vi "Multi-Record Stream Control.vi"(0 "actual state from slave":T1, 1 "ready to restart":bool, 2 "request state":T1, 3 "samples transferred":u64, 4 "num records":u64, 8 "reset":bool) -> (14 "request state to slave":T1, 15 "request to restart":bool, 16 "actual state":T1, 17 "total samples transferred":u64)   [LabVIEW 2018, in "Streaming FPGA.lvlib"]
doc: "Extends the <B>Acquisition Stream Control.vi</B> and the <B>Generation Stream Control.vi</B> with multi-record functionality.\n\nA finite transfer can be started by commanding the stream control VI from the \"Idle\" state to the \"Finite Transfer\" state. After the specified number of samples are transferred, the stream control VI enters the \"Done\" state. This multi-record stream control VI controls and monitors the state of a stream control VI to repeat the finite transfer <B>num records</B> times.\n\nThe <B>request state</B> input of this VI should receive the desired state of the multi-record stream control and the <B>request state to slave</B> output of this VI should drive the <B>request state</B> input of the stream control (<B>Acquisition Stream Control.vi</B> or <B>Generation Stream Control.vi</B>). Connect the <B>actual state</B> and <B>samples transferred</B> outputs of the stream control to the <B>actual state from slave</B> and <B>samples transferred</B> inputs of this VI through a Feedback Node. The <B>actual state</B> output of this VI returns the state of the multi-record stream control while the <B>total samples transferred</B> returns the total number of samples transferred since the multi-record transfer was started.\n\nCommanding the multi-record stream control from the \"Idle\" to the \"Finite Transfer\" state starts the multi-record transfer of <B>num records</B> records. For each record, the stream control is commanded from the \"Idle\" to the \"Finite Transfer\" state. When the stream control enters the \"Done\" state (signaling that the finite transfer is complete) and there are more records, the <B>request to restart</B> output is set to true for one cycle and the stream control is commanded into the \"Idle\" state, and a wait of 4 clock cycles starts. Once the wait is complete and the stream control enters the \"Idle\" state and a true is detected on the <B>ready to restart</B> input, the transfer of the next record starts by commanding the stream control from the \"Idle\" to the \"Finite Transfer\" state. During the multi-record transfer the <B>actual state</B> output returns \"Finite Transfer\" if the stream control indicates normal operation. If the stream control indicates an error or if a different state is requested on the <B>request state</B> input, then the multi-record transfer stops. When the stream control enters the \"Done\" state (signaling that the finite transfer is complete) and there are no more records, this VI also enters the \"Done\" state.\n\nWhen no multi-record transfer is in progress, the <B>request state to slave</B> output returns the <B>request state</B> input while the <B>actual state</B> and <B>total samples transferred</B> outputs return the <B>actual state from slave</B> and <B>samples transferred</B> inputs."
uses:
  Streaming FPGA.lvlib
  <instrlib>/_niInstr/Streaming/v1/Common/Stream State.ctl
  <instrlib>/_niInstr/Streaming/v1/Common/niInstr Streaming v1 Common.lvlib
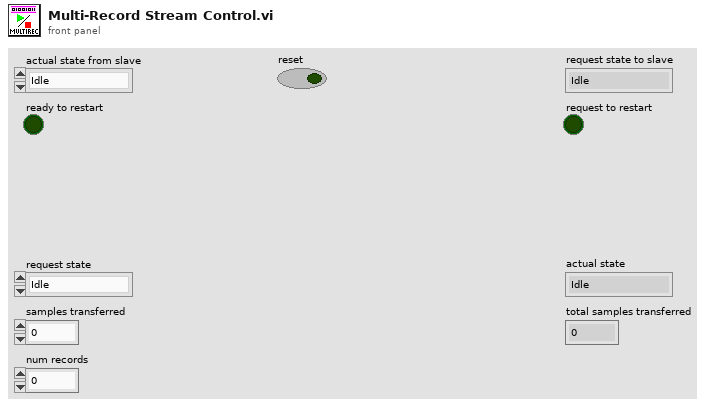
[diagram p1: front panel]
types:
  T1 = typedef "niInstr Streaming v1 Common.lvlib/Stream State.ctl" = enum8{"Idle", "Finite Transfer", "Continuous", "Done", "Error", "Not Ready", "Cancel"}
  T2 = enum16{"Idle", "Start Record", "Wait For Done", "Wait For Idle"}
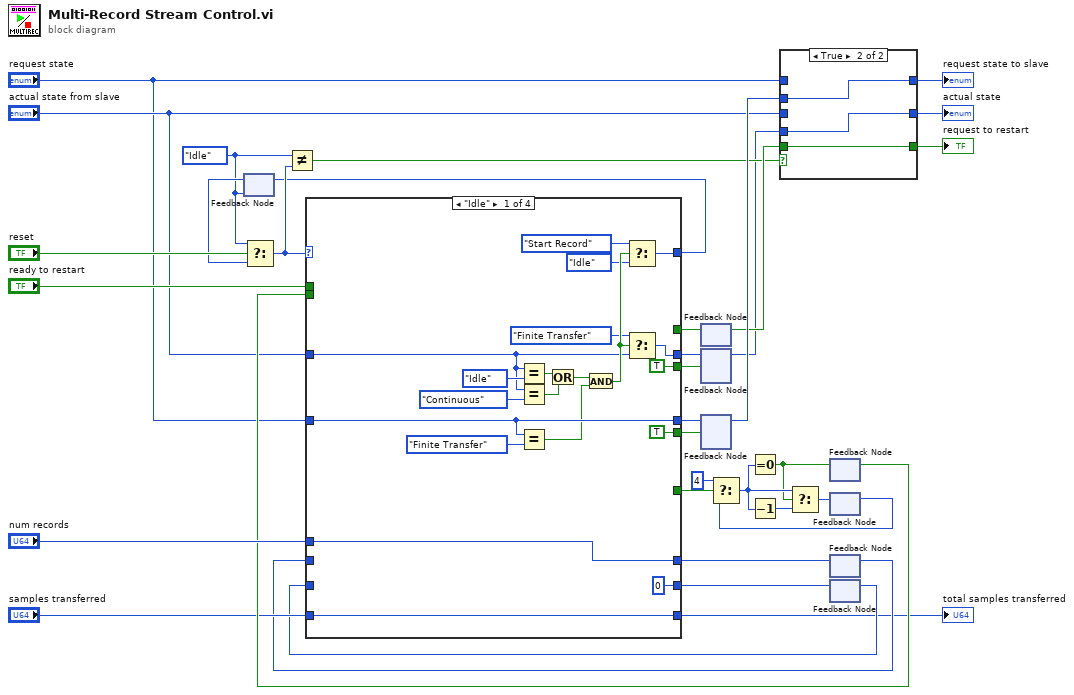
[diagram p0: block diagram]
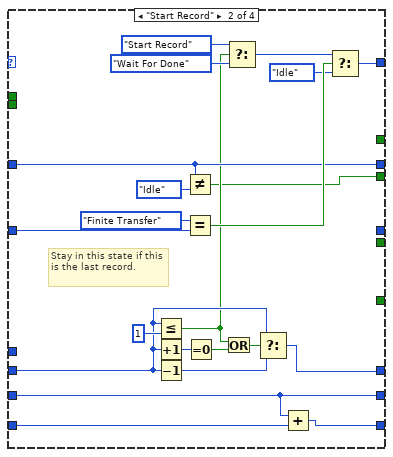
[diagram p2: hidden frame]
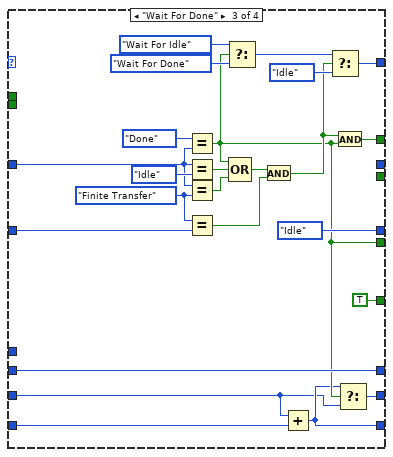
[diagram p3: hidden frame]
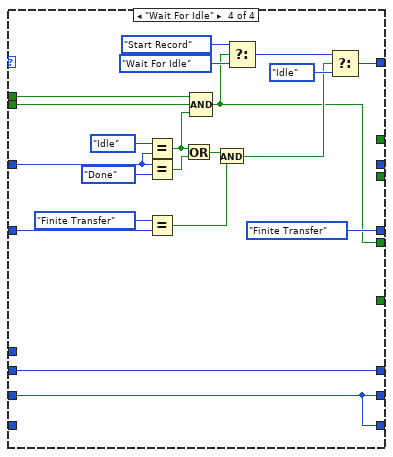
[diagram p4: hidden frame]
diagram:
  w24 = T2."Idle"
  n1 = feedback #1(w24) -> (w29:T2)
  n2 = Select(t=w24, s="reset", f=w29) -> (s? t:f=w25:T2)
  n3 = Not Equal?(x=w24, y=w25) -> (x != y?=w23:bool)
  n4 = feedback #2() -> (w31:bool)  [unwired: 1 in]
  n5 = feedback #3() -> (w7:T1)  [unwired: 1 in]
  n6 = feedback #4() -> (w32:T1)  [unwired: 1 in]
  n7 = case shown="True" w23 {
    tunnel: "actual state from slave" -> [w37 _]
    tunnel: [w37 w38] -> w34
    tunnel: [w36 w39] -> w33
    tunnel: w32 -> [_ w39]
    tunnel: w31 -> [_ w40]
    tunnel: [_ w40] -> w30
    tunnel: "request state" -> [w36 _]
    tunnel: w7 -> [_ w38]
    frame False {
    }
    frame True {
    }
  }
  "actual state" <- w34
  "request state to slave" <- w33
  "request to restart" <- w30
  n8 = feedback #5() -> (w17:bool)  [unwired: 1 in]
  n9 = feedback #6() -> (w14:u8)  [unwired: 1 in]
  n10 = feedback #7() -> (w4:u64)  [unwired: 1 in]
  n11 = feedback #8() -> (w3:u64)  [unwired: 1 in]
  n12 = case shown="\"Idle\"" w25 {
    tunnel: "num records" -> [w55 _ _ _]
    tunnel: "ready to restart" -> [_ _ _ w115]
    tunnel: "request state" -> [w54 w73 w93 w120]
    tunnel: "actual state from slave" -> [w45 w67 w96 w121]
    tunnel: [w54 _ Stream_State."Idle" ("y") Stream_State."Finite Transfer" ("request state")] -> w26
    tunnel: [w56 w69 w102 w112] -> w22
    tunnel: w4 -> [_ w78 w101 w117]
    tunnel: [w55 w76 w101 w117] -> w5
    tunnel: [_ _ w97 _] -> w21
    tunnel: [_ _ TRUE _] -> w20
    tunnel: w17 -> [_ _ _ w114]
    tunnel: [TRUE _ w86 w108] -> w18
    tunnel: [w44 w67 _ _] -> w9
    tunnel: [TRUE w64 _ _] -> w8
    tunnel: "samples transferred" -> [w41 w63 w87 _]
    tunnel: w3 -> [_ w61 w83 w107]
    tunnel: [u64 0 w61 w85 w107] -> w2
    tunnel: [w41 w62 w84 w107] -> w1
    frame "Idle" {
      n13 = Equal?(x=w45, y=Stream_State."Idle" ("actual state from slave")) -> (x = y?=w48:bool)
      n14 = Equal?(x=w45, y=Stream_State."Continuous" ("actual state from slave")) -> (x = y?=w49:bool)
      n15 = Equal?(x=w54, y=Stream_State."Finite Transfer" ("x")) -> (x = y?=w46:bool)
      n16 = Or(x=w48, y=w49) -> (x .or. y?=w47:bool)
      n17 = And(x=w47, y=w46) -> (x .and. y?=w60:bool)
      n18 = Select(t=T2."Start Record", s=w60, f=T2."Idle") -> (s? t:f=w56:T2)
      n19 = Select(t=Stream_State."Finite Transfer", s=w60, f=w45) -> (s? t:f=w44:T1)
    }
    frame "Start Record" {
      # "Stay in this state if this is the last record."
      n20 = Less Or Equal?(x=w78, y=u64 1) -> (x <= y?=w65:bool)
      n21 = Increment(x=w78) -> (x+1=w80:u64)
      n22 = Decrement(x=w78) -> (x-1=w77:u64)
      n23 = Not Equal?(x=w67, y=Stream_State."Idle") -> (x != y?=w64:bool)
      n24 = Equal?(x=Stream_State."Finite Transfer", y=w73) -> (x = y?=w82:bool)
      n25 = Equal To 0?(x=w80) -> (x = 0?=w79:bool)
      n26 = Or(x=w65, y=w79) -> (x .or. y?=w68:bool)
      n27 = Select(t=T2."Start Record", s=w65, f=T2."Wait For Done") -> (s? t:f=w71:T2)
      n28 = Select(t=w78, s=w68, f=w77) -> (s? t:f=w76:u64)
      n29 = Add(x=w61, y=w63) -> (x+y=w62:u64)
      n30 = Select(t=w71, s=w82, f=T2."Idle") -> (s? t:f=w69:T2)
    }
    frame "Wait For Done" {
      w92 = Stream_State."Finite Transfer" ("y")
      n31 = Equal?(x=Stream_State."Done" ("y"), y=w96) -> (x = y?=w86:bool)
      n32 = Equal?(x=w96, y=Stream_State."Idle") -> (x = y?=w90:bool)
      n33 = Equal?(x=w96, y=w92) -> (x = y?=w91:bool)
      n34 = Equal?(x=w92, y=w93) -> (x = y?=w104:bool)
      n35 = Select(t=T2."Wait For Idle", s=w86, f=T2."Wait For Done") -> (s? t:f=w100:T2)
      n36 = Compound Arithmetic op=OR(w86, w90, w91) -> (w105:bool)
      n37 = And(x=w105, y=w104) -> (x .and. y?=w94:bool)
      n38 = Add(x=w83, y=w87) -> (x+y=w84:u64)
      n39 = Select(t=w100, s=w94, f=T2."Idle") -> (s? t:f=w102:T2)
      n40 = And(x=w94, y=w86) -> (x .and. y?=w97:bool)
      n41 = Select(t=w84, s=w86, f=w83) -> (s? t:f=w85:u64)
    }
    frame "Wait For Idle" {
      n42 = Equal?(x=Stream_State."Idle" ("y"), y=w121) -> (x = y?=w111:bool)
      n43 = Equal?(x=w121, y=Stream_State."Done" ("x")) -> (x = y?=w116:bool)
      n44 = Equal?(x=Stream_State."Finite Transfer" ("y"), y=w120) -> (x = y?=w119:bool)
      n45 = Or(x=w111, y=w116) -> (x .or. y?=w118:bool)
      n46 = Compound Arithmetic op=AND(w115, w114, w111) -> (w108:bool)
      n47 = And(x=w118, y=w119) -> (x .and. y?=w109:bool)
      n48 = Select(t=T2."Start Record", s=w108, f=T2."Wait For Idle") -> (s? t:f=w113:T2)
      n49 = Select(t=w113, s=w109, f=T2."Idle") -> (s? t:f=w112:T2)
    }
  }
  "total samples transferred" <- w1
  n50 = feedback-in #1(w22) -> ()
  n51 = feedback-in #2(w21) -> ()
  n52 = feedback-in #3(w9, w8) -> ()
  n53 = feedback-in #4(w26, w18) -> ()
  n54 = Select(t=u8 4, s=w20, f=w14) -> (s? t:f=w13:u8)
  n55 = Equal To 0?(x=w13) -> (x = 0?=w12:bool)
  n56 = Decrement(x=w13) -> (x-1=w16:u8)
  n57 = Select(t=w13, s=w12, f=w16) -> (s? t:f=w15:u8)
  n58 = feedback-in #5(w12) -> ()
  n59 = feedback-in #6(w15) -> ()
  n60 = feedback-in #7(w5) -> ()
  n61 = feedback-in #8(w2) -> ()
